vi "Property.vi"() -> ()   [LabVIEW 2012]
panel:
  in  "ICImagingControl":refnum<k7>(container)
  out "Picture Out":picture
  in  "Open Device Configuration (Monochrome  Images)":bool
  in  "Open Device Configuration (Color Images)":bool
  in  "Automatic":bool
  in  "Value":i32(slide) caption="Sharpness" scale=-11.0..-5.0
  in  "Properties":i32(listbox)
  out "Property Array":T1(array[ring])
  in  "Grab":bool
  in  "End Program":bool
  # "Open Device Configuration"
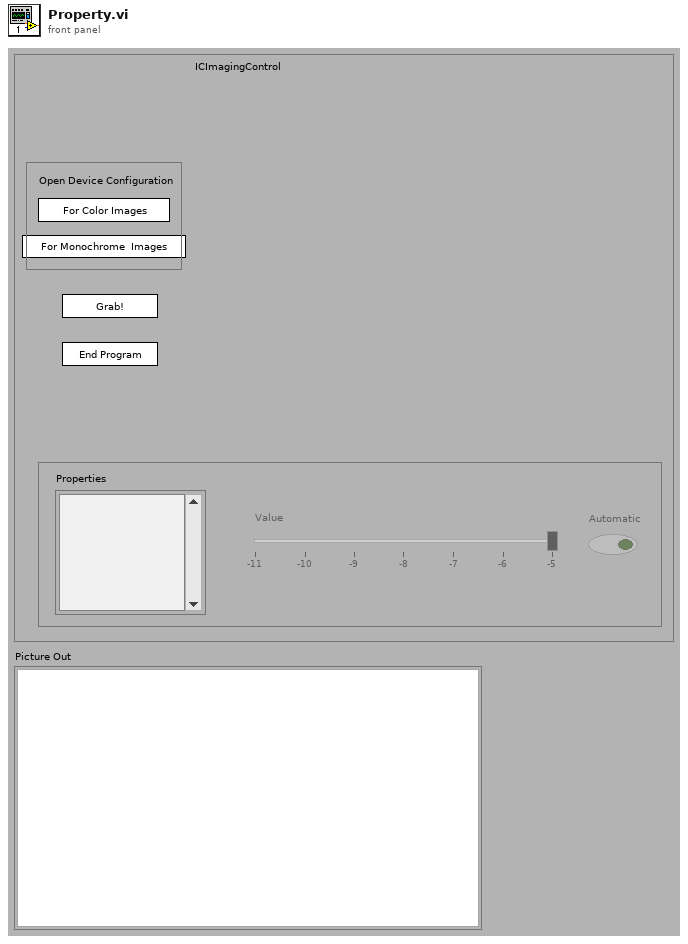
[diagram p1: front panel]
types:
  T1 = enum16{"Brightness", "Color Enable", "Contrast", "Exposure", "Focus", "Gain", "Gamma", "Hue", "Iris", "Pan", "Roll", "Saturation", "Sharpness", "Tilt", "Whitebalance", "Zoom", "Whitebalance Blue", "Whitebalance Red"}[]
  T2 = enum16{"Brightness", "Color Enable", "Contrast", "Exposure", "Focus", "Gain", "Gamma", "Hue", "Iris", "Pan", "Roll", "Saturation", "Sharpness", "Tilt", "Whitebalance", "Zoom", "Whitebalance Blue", "Whitebalance Red"}
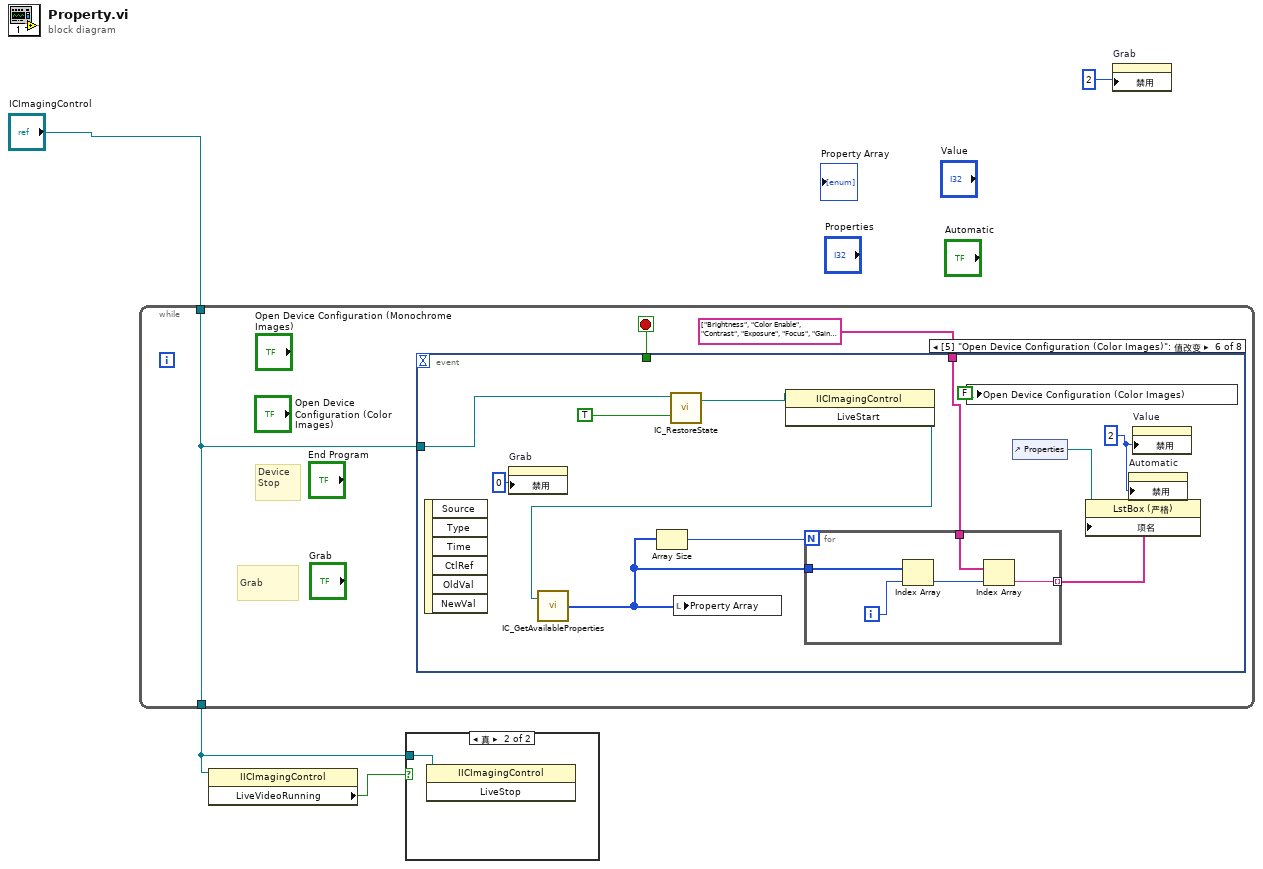
[diagram p0: block diagram]
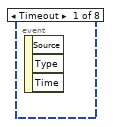
[diagram p3: hidden frame]
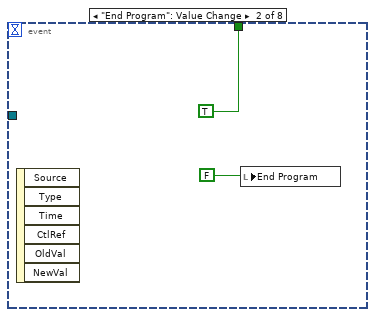
[diagram p4: hidden frame]
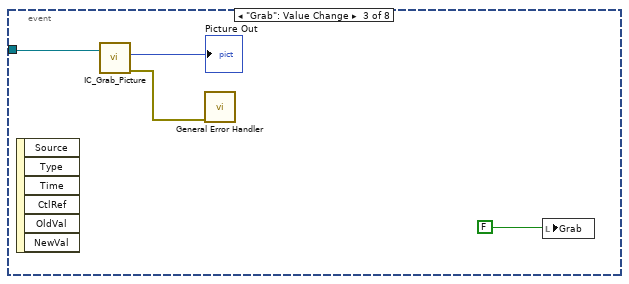
[diagram p5: hidden frame]
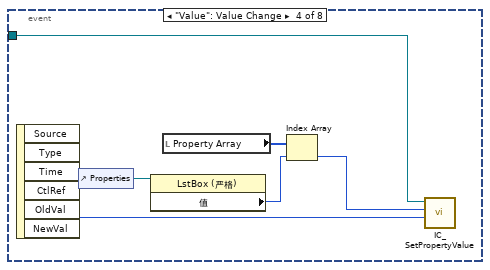
[diagram p6: hidden frame]
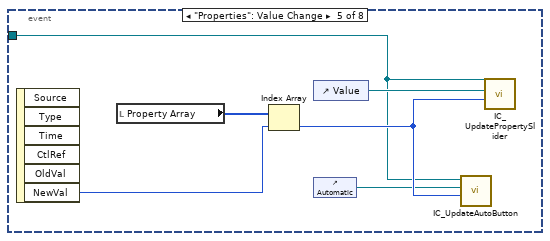
[diagram p7: hidden frame]
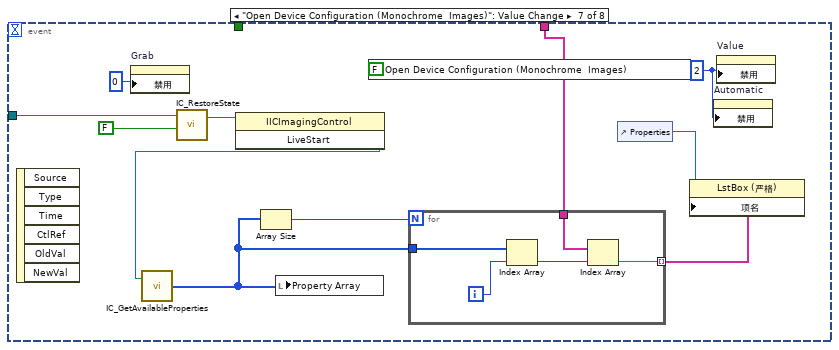
[diagram p8: hidden frame]
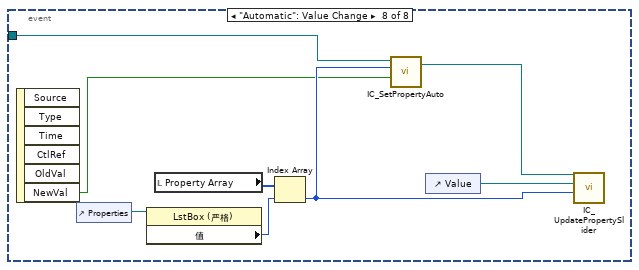
[diagram p9: hidden frame]
diagram:
  n1 = while {
    tunnel: "ICImagingControl" -> [w6]
    tunnel: [w6] -> w3
    stop <- w7 stop-if-true
    # "Device\nStop"
    # "Grab"
    n2 = event shown="[5] \"Open Device Configuration (Color Images)\": 值改变" {
      selector: _ -> [_ _ _ _ _ _ _ _]
      dyn-events: _ -> [_ _ _ _ _ _ _ _]
      timeout: _ -> [_ _ _ _ _ _ _ _]
      tunnel: w6 -> [_ _ w11 w16 w20 w29 w46 w63]
      tunnel: [_ TRUE _ _ _ _ _ _] -> w7
      tunnel: string[] ["Brightness", "Color Enable", "Contrast", "Exposure", "Focus", "Gain", "Gamma", "Hue", "Iris", "Pan", "Roll", "Saturation", "Sharpness", "Tilt", "Whitebalance", "Zoom", "Whitebalance Blue", "Whitebalance Red"] ("Item Names") -> [_ _ _ _ _ w27 w44 _]
      event Timeout {
        n3 = event-data() -> ()  [unwired: 1 in, 3 out]
      }
      event "End Program": Value Change {
        n4 = event-data() -> ()  [unwired: 1 in, 6 out]
        n5 = local write "End Program"(FALSE) -> ()
      }
      event "Grab": Value Change {
        n6 = event-data() -> ()  [unwired: 1 in, 6 out]
        n7 = call "IC_Grab_Picture.vi"("ICImagingControl In"=w11) -> ("Picture Out"=→"Picture Out":picture, "Error Out"=w12:errorcluster)  [unwired: 1 in, 2 out]
        n8 = call <vilib>:"General Error Handler.vi"("error in (no error)"=w12) -> ()  [unwired: 10 in, 5 out]
        n9 = local write "Grab"(FALSE) -> ()
      }
      event "Value": Value Change {
        n10 = event-data() -> ("NewVal"=w14:i32)  [unwired: 1 in, 5 out]
        n11 = control-ref of="Properties"() -> (w17:refnum<vi>)
        n12 = property class="LstBox (严格)"(reference=w17) -> ("值"=w18:i32)  [unwired: 1 in, 2 out]
        n13 = local read "Property Array"() -> (w19:T1)
        n14 = Index Array(array=w19, index=w18) -> (element=w15:T2)
        n15 = call <userlib>:"IC_SetPropertyValue.vi"("Value"=w14, "Property"=w15, "ICImagingControl In"=w16) -> ()  [unwired: 1 in, 2 out]
      }
      event "Properties": Value Change {
        n16 = event-data() -> ("NewVal"=w24:i32)  [unwired: 1 in, 5 out]
        n17 = local read "Property Array"() -> (w25:T1)
        n18 = Index Array(array=w25, index=w24) -> (element=w22:T2)
        n19 = control-ref of="Value"() -> (w23:refnum<vi>)
        n20 = control-ref of="Automatic"() -> (w21:refnum<vi>)
        n21 = call <userlib>:"IC_UpdateAutoButton.vi"("Property"=w22, "Button"=w21, "ICImagingControl In"=w20) -> ()  [unwired: 1 in, 2 out]
        n22 = call <userlib>:"IC_UpdatePropertySlider.vi"("Property"=w22, "Slider"=w23, "ICImagingControl In"=w20) -> ()  [unwired: 1 in, 2 out]
      }
      event "Open Device Configuration (Color Images)": Value Change {
        w28 = 2
        n23 = event-data() -> ()  [unwired: 1 in, 6 out]
        n24 = property on="Grab" class="Bool (严格)"("禁用"=u8 0 ("Disabled")) -> ()  [unwired: 2 in, 2 out]
        n25 = call "IC_RestoreState.vi"("Color"=TRUE, "ICImagingControl"=w29) -> ("ICImagingControl Out"=w36:refnum<k7>)  [unwired: 2 in, 1 out]
        n26 = invoke class="IICImagingControl" method="LiveStart"(reference=w36) -> (reference out=w26:refnum<k7>)  [unwired: 2 in, 2 out]
        n27 = call <userlib>:"IC_GetAvailableProperties.vi"("ICImagingControl In"=w26) -> ("Properties"=w31:T1)  [unwired: 1 in, 2 out]
        n28 = Array Size(array=w31) -> (size(s)=w32:i32)
        n29 = local write "Property Array"(w31) -> ()
        n30 = for {
          N: w32 -> [_]
          tunnel: [w42] -> w33 mode=indexing
          tunnel: w27 -> [w41]
          tunnel: w31 -> [w39]
          i -> [w38]
          n31 = Index Array(array=w39, index=w38) -> (element=w40:T2)
          n32 = Index Array(array=w41, index=w40) -> (element=w42:string)
        }
        n33 = local write "Open Device Configuration (Color Images)"(FALSE) -> ()
        n34 = control-ref of="Properties"() -> (w30:refnum<vi>)
        n35 = property class="LstBox (严格)"(reference=w30, "项名"=w33) -> ()  [unwired: 1 in, 2 out]
        n36 = property on="Automatic" class="Bool (严格)"("禁用"=w28) -> ()  [unwired: 2 in, 2 out]
        n37 = property on="Value" class="Slide (严格)"("禁用"=w28) -> ()  [unwired: 2 in, 2 out]
      }
      event "Open Device Configuration (Monochrome  Images)": Value Change {
        w45 = 2
        n38 = event-data() -> ()  [unwired: 1 in, 6 out]
        n39 = property on="Grab" class="Bool (严格)"("禁用"=0) -> ()  [unwired: 2 in, 2 out]
        n40 = call "IC_RestoreState.vi"("Color"=FALSE, "ICImagingControl"=w46) -> ("ICImagingControl Out"=w52:refnum<k7>)  [unwired: 2 in, 1 out]
        n41 = invoke class="IICImagingControl" method="LiveStart"(reference=w52) -> (reference out=w43:refnum<k7>)  [unwired: 2 in, 2 out]
        n42 = call <userlib>:"IC_GetAvailableProperties.vi"("ICImagingControl In"=w43) -> ("Properties"=w48:T1)  [unwired: 1 in, 2 out]
        n43 = Array Size(array=w48) -> (size(s)=w49:i32)
        n44 = local write "Property Array"(w48) -> ()
        n45 = local write "Open Device Configuration (Monochrome  Images)"(FALSE ("Open Device Configuration (Monochrome  Images)")) -> ()
        n46 = for {
          N: w49 -> [_]
          tunnel: [w59] -> w50 mode=indexing
          tunnel: w44 -> [w58]
          tunnel: w48 -> [w56]
          i -> [w55]
          n47 = Index Array(array=w56, index=w55) -> (element=w57:T2)
          n48 = Index Array(array=w58, index=w57) -> (element=w59:string)
        }
        n49 = control-ref of="Properties"() -> (w47:refnum<vi>)
        n50 = property class="LstBox (严格)"(reference=w47, "项名"=w50) -> ()  [unwired: 1 in, 2 out]
        n51 = property on="Automatic" class="Bool (严格)"("禁用"=w45) -> ()  [unwired: 2 in, 2 out]
        n52 = property on="Value" class="Slide (严格)"("禁用"=w45) -> ()  [unwired: 2 in, 2 out]
      }
      event "Automatic": Value Change {
        n53 = event-data() -> ("NewVal"=w60:bool)  [unwired: 1 in, 5 out]
        n54 = control-ref of="Properties"() -> (w65:refnum<vi>)
        n55 = property class="LstBox (严格)"(reference=w65) -> ("值"=w67:i32)  [unwired: 1 in, 2 out]
        n56 = local read "Property Array"() -> (w66:T1)
        n57 = Index Array(array=w66, index=w67) -> (element=w62:T2)
        n58 = call <userlib>:"IC_SetPropertyAuto.vi"("Auto"=w60, "Property"=w62, "ICImagingControl In"=w63) -> ("ICImagingControl Out"=w61:refnum<k7>)  [unwired: 1 in, 1 out]
        n59 = control-ref of="Value"() -> (w64:refnum<vi>)
        n60 = call <userlib>:"IC_UpdatePropertySlider.vi"("Property"=w62, "Slider"=w64, "ICImagingControl In"=w61) -> ()  [unwired: 1 in, 2 out]
      }
    }
  }
  n61 = property class="IICImagingControl"(reference=w3) -> ("LiveVideoRunning"=w4:bool)  [unwired: 1 in, 2 out]
  n62 = case shown="真" w4 {
    tunnel: w3 -> [_ w68]
    frame False {
    }
    frame True {
      n63 = invoke class="IICImagingControl" method="LiveStop"(reference=w68) -> ()  [unwired: 2 in, 3 out]
    }
  }
  n64 = property on="Grab" class="Bool (严格)"("禁用"=2) -> ()  [unwired: 2 in, 2 out]
